vi "load_parameters_csv.vi"(8 "error in (no error)":errorcluster, 10 "Parameter CSV Path":string, 11 "Tags In":string) -> (0 "error out":errorcluster, 1 "Computer Found":bool, 2 "Loaded Params":string[][](array[string]), 3 "Parameters Out":T1)   [LabVIEW 2019]
uses:
  Parameters.ctl
  <vilib>/Utility/file.llb/Read Delimited Spreadsheet (string).vi
panel:
  in  "Parameters":T1
  # "Faux Worm Drawing"
  # "Tracking"
  # "Temporal Calibration"
  # "Stimulus Generation"
  # "Median Filtering"
  # "Experimental Settings"
  # "Camera and Projector Settings"
  # "Faux Worm Drawing"
  # "Tracking"
  # "Temporal Calibration"
  # "Stimulus Generation"
  # "Median Filtering"
  # "Experimental Settings"
  # "Camera and Projector Settings"
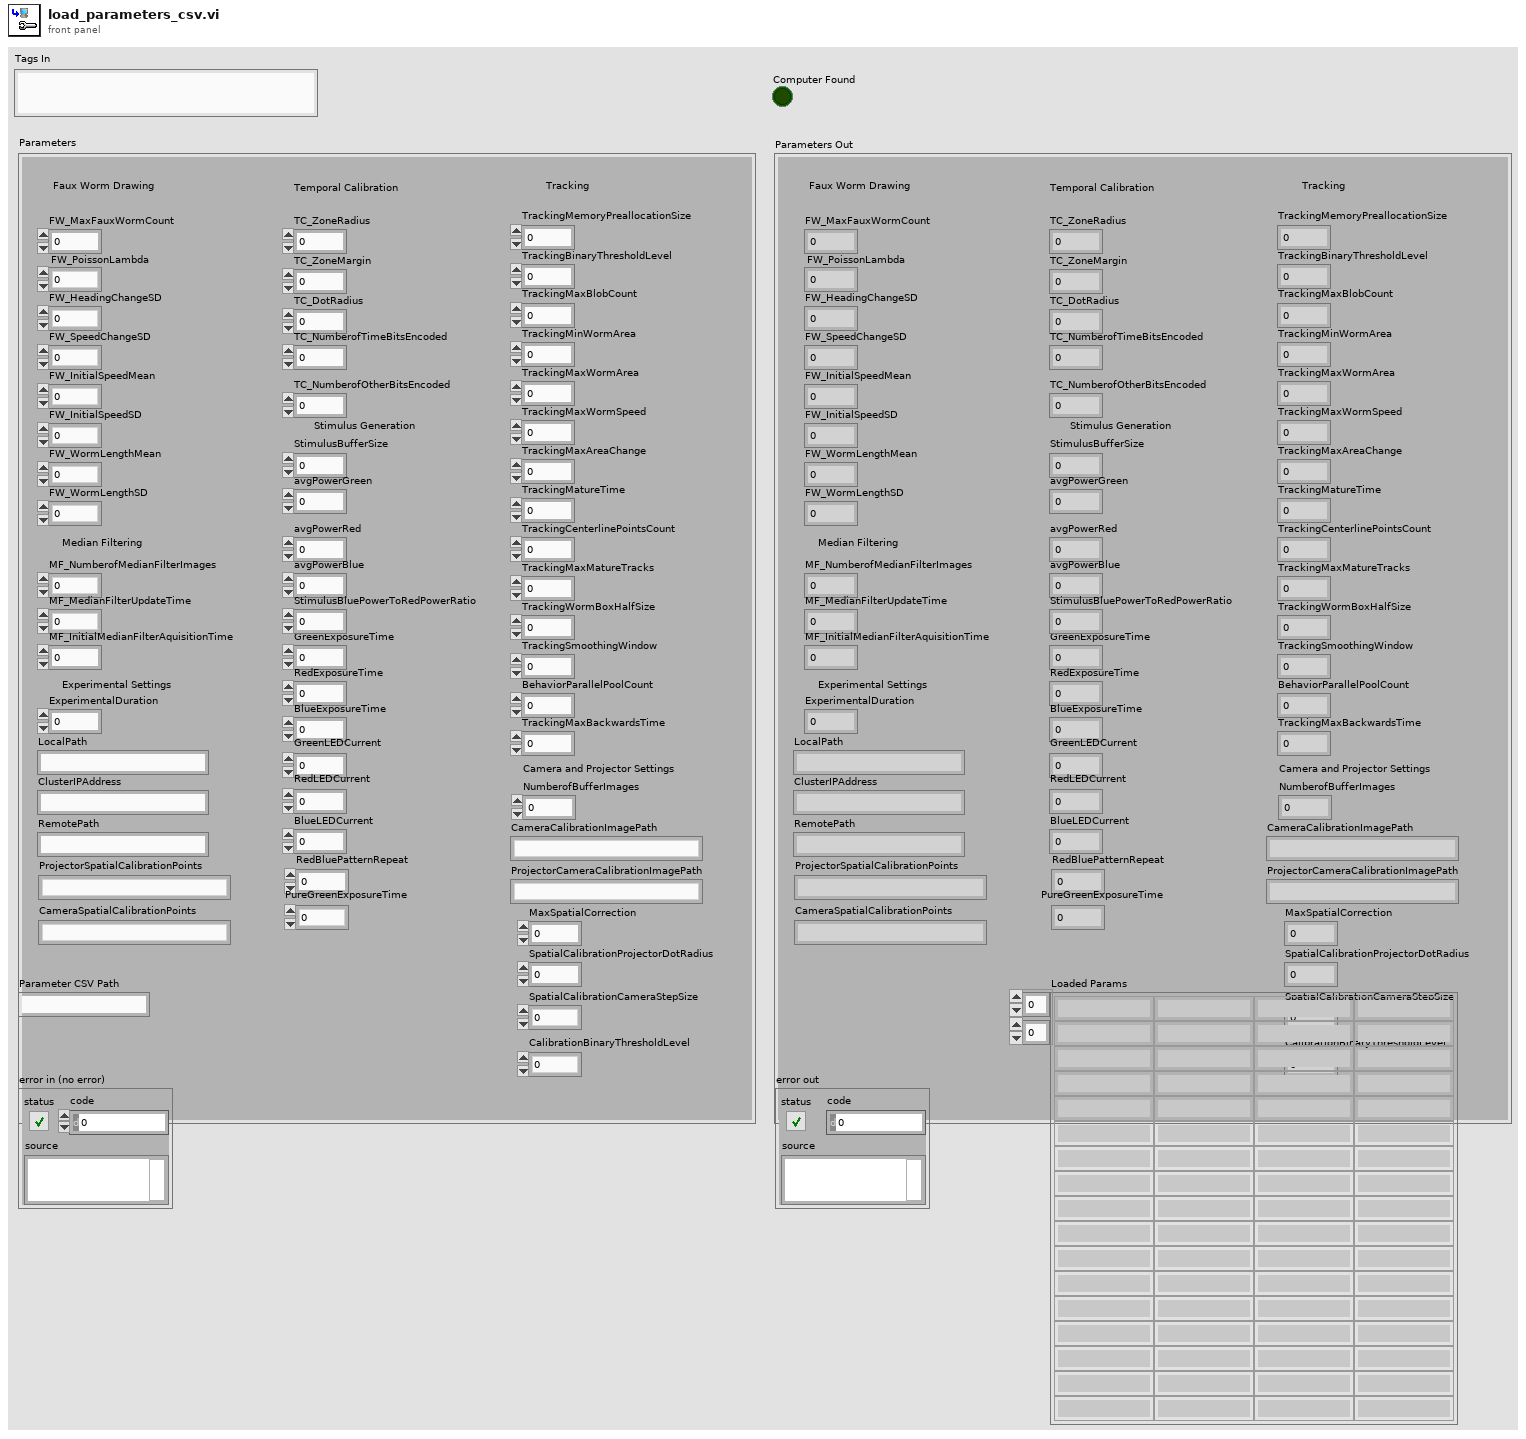
[diagram p1: front panel]
types:
  T1 = typedef "Parameters.ctl" = cluster{"FW_MaxFauxWormCount":i32, "FW_PoissonLambda":dbl, "FW_HeadingChangeSD":dbl, "FW_SpeedChangeSD":dbl, "FW_InitialSpeedMean":dbl, "FW_InitialSpeedSD":dbl, "FW_WormLengthMean":dbl, "FW_WormLengthSD":dbl, "MF_NumberofMedianFilterImages":i32, "MF_MedianFilterUpdateTime":i32, "MF_InitialMedianFilterAquisitionTime":dbl, "ExperimentalDuration":i32, "TC_ZoneRadius":i32, "TC_ZoneMargin":i32, "TC_DotRadius":dbl, "TC_NumberofTimeBitsEncoded":i32, "TC_NumberofOtherBitsEncoded":i32, "NumberofBufferImages":sgl, "CameraCalibrationImagePath":string, "ProjectorCameraCalibrationImagePath":string, "StimulusBufferSize":i32, "TrackingMemoryPreallocationSize":i32, "TrackingBinaryThresholdLevel":sgl, "TrackingMaxBlobCount":i32, "TrackingMinWormArea":dbl, "TrackingMaxWormArea":dbl, "TrackingMaxWormSpeed":dbl, "TrackingMaxAreaChange":dbl, "TrackingMatureTime":i32, "TrackingCenterlinePointsCount":i32, "TrackingMaxMatureTracks":i32, "TrackingWormBoxHalfSize":i32, "TrackingSmoothingWindow":i32, "BehaviorParallelPoolCount":i32, "LocalPath":string, "GreenExposureTime":i32, "RedExposureTime":i32, "BlueExposureTime":i32, "ClusterIPAddress":string, "RemotePath":string, "GreenLEDCurrent":u8, "RedLEDCurrent":u8, "BlueLEDCurrent":u8, "avgPowerGreen":sgl, "avgPowerRed":sgl, "avgPowerBlue":sgl, "StimulusBluePowerToRedPowerRatio":sgl, "TrackingMaxBackwardsTime":i32, "MaxSpatialCorrection":dbl, "ProjectorSpatialCalibrationPoints":string, "SpatialCalibrationProjectorDotRadius":i32, "SpatialCalibrationCameraStepSize":dbl, "CameraSpatialCalibrationPoints":string, "CalibrationBinaryThresholdLevel":dbl, "RedBluePatternRepeat":i32, "PureGreenExposureTime":i32}
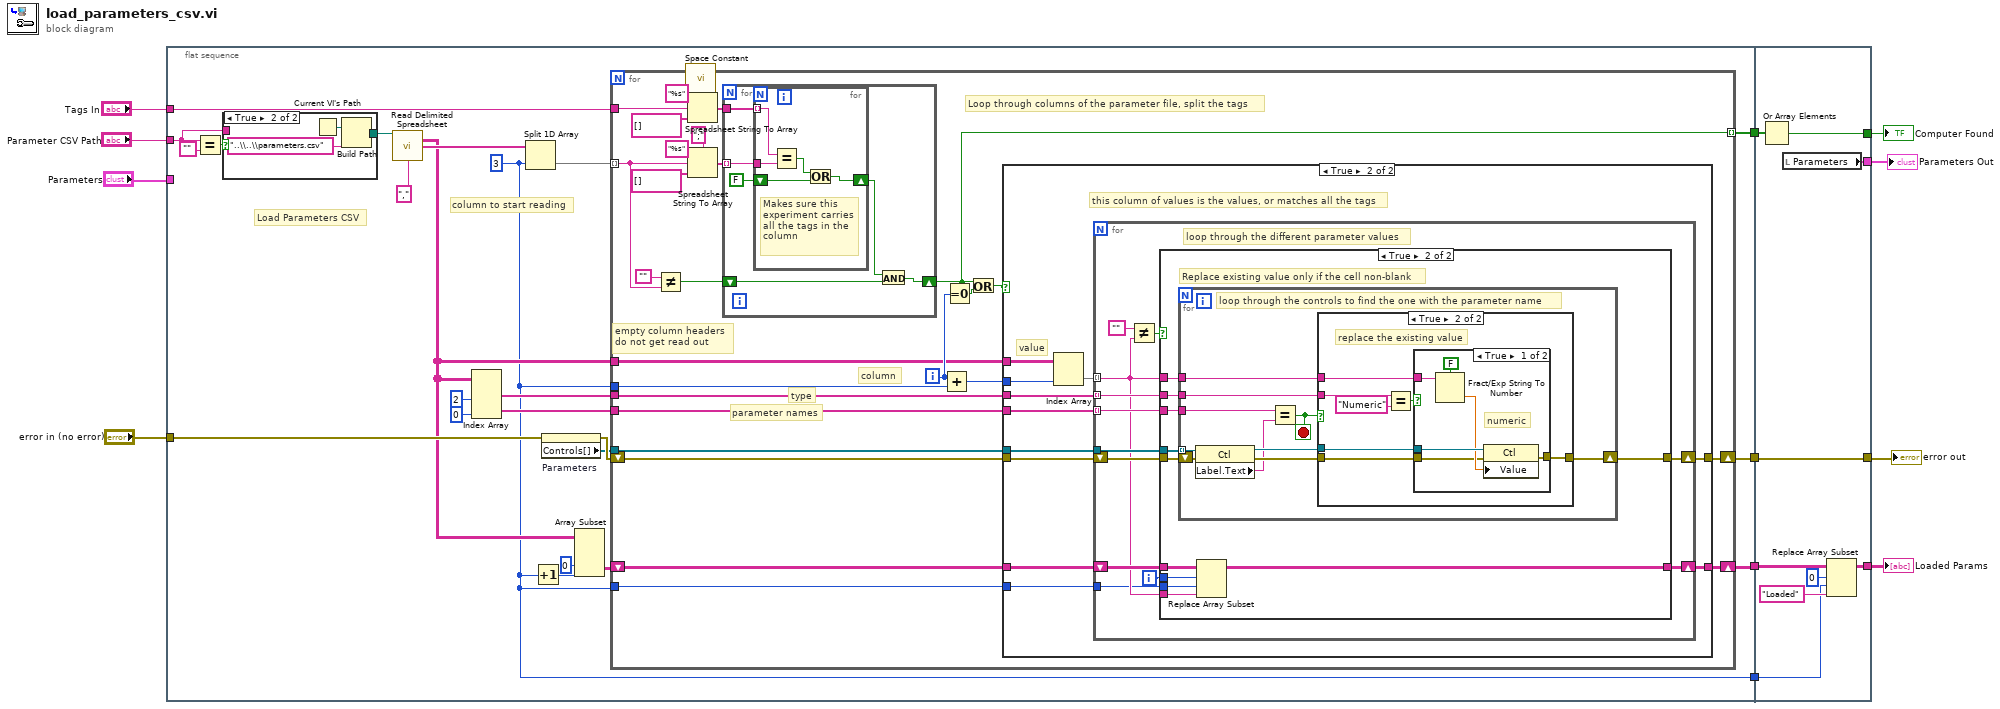
[diagram p0: block diagram]
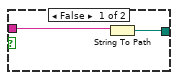
[diagram p2: hidden frame]
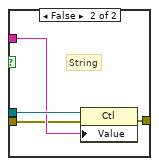
[diagram p6: hidden frame]
diagram:
  n1 = flat-sequence {
    tunnel: "error in (no error)" -> [w25]
    tunnel: [w24] -> w11
    tunnel: "Parameters" -> [_]
    tunnel: "Tags In" -> [w23]
    tunnel: [w19] -> w6
    tunnel: [w17] -> w4
    tunnel: "Parameter CSV Path" -> [w14]
    tunnel: [w13] -> w2
    tunnel: w11 -> [w152]
    tunnel: [w153] -> w10
    tunnel: [w152] -> w9
    tunnel: w6 -> [w149]
    tunnel: [w148] -> w5
    tunnel: w4 -> [w147]
    tunnel: w2 -> [w146]
    tunnel: [w145] -> w1
    frame #0 {
      w17 = 3 ("y")
      # "column to start reading"
      # "Load Parameters CSV"
      n2 = Equal?(x=w14, y="") -> (x = y?=w15:bool)
      n3 = case shown="True" w15 {
        tunnel: [w37 w39] -> w35
        tunnel: w14 -> [w36 _]
        frame False {
          n4 = String To Path(string=w36) -> (path=w37:path)
        }
        frame True {
          n5 = Current VI's Path() -> (path=w40:path)
          n6 = Build Path(base path=w40, name or relative path="..\\..\\parameters.csv") -> (appended path=w39:path)
        }
      }
      n7 = call-poly <vilib>:"Read Delimited Spreadsheet.vi"("file path (dialog if empty)"=w35, "delimiter (\\t)"=",") -> ("all rows"=w18:string[][], "first row"=w27:string[])  [unwired: 8 in, 4 out]
      n8 = Index Array(array=w18, index (col) #1=2 ("disabled index (col)"), index (col) #2=0 ("index (col)")) -> (element #1=w32:string[], element #2=w30:string[])  [unwired: 2 in]
      n9 = Split 1D Array(array=w27, index=w17) -> (second subarray=w26:string[])  [unwired: 1 out]
      n10 = Increment(x=w17) -> (x+1=w21:i32)
      n11 = property on="Parameters" class="Clust (strict)"(error in=w25) -> (error out=w29:errorcluster, "Controls[]"=w28:refnum<vi>[])  [unwired: 1 in, 1 out]
      n12 = Array Subset(array=w18, index (col)=0 ("index"), length (col)=w21) -> (w20:string[][])  [unwired: 2 in]
      n13 = for {
        tunnel: w23 -> [w67]
        tunnel: w26 -> [w46] mode=indexing
        tunnel: w32 -> [w55]
        tunnel: w30 -> [w54]
        tunnel: w18 -> [w53]
        tunnel: w28 -> [w51]
        shift-right: [w49] -> w24
        shift-left: w29 -> [w50]
        tunnel: w17 -> [w48]
        shift-right: [w43] -> w19
        shift-left: w20 -> [w44]
        tunnel: w17 -> [w42]
        tunnel: [w41] -> w13 mode=indexing
        i -> [w58]
        # "empty column headers\ndo not get read out"
        # "type"
        # "parameter names"
        # "column"
        # "Loop through columns of the parameter file, split the tags"
        n14 = Not Equal?(x="", y=w46) -> (x != y?=w45:bool)
        n15 = call <vilib>:"Space Constant.vi"() -> ("String"=w59:string)
        n16 = Spreadsheet String To Array(delimiter (Tab)=w59, format string="%s", spreadsheet string=w67, array type (2D Dbl)=string[] []) -> (array=w64:string[])
        n17 = Spreadsheet String To Array(delimiter (Tab)=";", format string="%s", spreadsheet string=w46, array type (2D Dbl)=string[] []) -> (array=w61:string[])
        n18 = for {
          tunnel: w64 -> [w139]
          tunnel: w61 -> [w138] mode=indexing
          shift-right: [w136] -> w41
          shift-left: w45 -> [w134]
          n19 = for {
            tunnel: w139 -> [w144] mode=indexing
            tunnel: w138 -> [w143]
            shift-right: [w140] -> w135
            shift-left: FALSE -> [w141]
            # "Makes sure this\nexperiment carries\nall the tags in the\ncolumn"
            n20 = Equal?(x=w144, y=w143) -> (x = y?=w142:bool)
            n21 = Or(x=w142, y=w141) -> (x .or. y?=w140:bool)
          }
          n22 = And(x=w135, y=w134) -> (x .and. y?=w136:bool)
        }
        n23 = Add(x=w58, y=w48) -> (x+y=w52:i32)
        n24 = Equal To 0?(x=w58) -> (x = 0?=w57:bool)
        n25 = Or(x=w41, y=w57) -> (x .or. y?=w56:bool)
        n26 = case shown="True" w56 {
          tunnel: w55 -> [_ w77]
          tunnel: w54 -> [_ w76]
          tunnel: w53 -> [_ w80]
          tunnel: w52 -> [_ w79]
          tunnel: w51 -> [_ w75]
          tunnel: w50 -> [w69 w74]
          tunnel: [w69 w73] -> w49
          tunnel: w44 -> [w68 w72]
          tunnel: [w68 w70] -> w43
          tunnel: w42 -> [_ w71]
          frame False {
          }
          frame True {
            # "this column of values is the values, or matches all the tags"
            # "value"
            n27 = Index Array(array=w80, index (col)=w79) -> (element=w78:string[])  [unwired: 1 in]
            n28 = for {
              tunnel: w78 -> [w83] mode=indexing
              tunnel: w77 -> [w89] mode=indexing
              tunnel: w76 -> [w88] mode=indexing
              tunnel: w75 -> [w90]
              shift-right: [w86] -> w73
              shift-left: w74 -> [w87]
              shift-right: [w84] -> w70
              shift-left: w72 -> [w85]
              tunnel: w71 -> [w82]
              i -> [w81]
              # "loop through the different parameter values"
              n29 = Not Equal?(x="", y=w83) -> (x != y?=w91:bool)
              n30 = case shown="True" w91 {
                tunnel: w90 -> [_ w105]
                tunnel: w89 -> [_ w104]
                tunnel: w88 -> [_ w103]
                tunnel: w83 -> [_ w102]
                tunnel: w87 -> [w94 w101]
                tunnel: [w94 w100] -> w86
                tunnel: w85 -> [w93 w99]
                tunnel: [w93 w95] -> w84
                tunnel: w83 -> [_ w96]
                tunnel: w82 -> [_ w98]
                tunnel: w81 -> [_ w97]
                frame False {
                }
                frame True {
                  # "Replace existing value only if the cell non-blank"
                  n31 = for {
                    tunnel: w105 -> [w114] mode=indexing
                    tunnel: w104 -> [w111]
                    tunnel: w103 -> [w115]
                    tunnel: w102 -> [w112]
                    shift-right: [w108] -> w100
                    shift-left: w101 -> [w110]
                    stop <- w107 stop-if-true
                    # "loop through the controls to find the one with the parameter name"
                    n32 = property class="Ctl"(reference=w114, error in=w110) -> (reference out=w113:refnum<vi>, error out=w109:errorcluster, "Label.Text"=w106:string)
                    n33 = Equal?(x=w115, y=w106) -> (x = y?=w107:bool)
                    n34 = case shown="True" w107 {
                      tunnel: w113 -> [_ w123]
                      tunnel: w112 -> [_ w119]
                      tunnel: w111 -> [_ w122]
                      tunnel: w109 -> [w116 w118]
                      tunnel: [w116 w117] -> w108
                      frame False {
                      }
                      frame True {
                        # "replace the existing value"
                        n35 = Equal?(x=w122, y="Numeric") -> (x = y?=w120:bool)
                        n36 = case shown="True" w120 {
                          tunnel: w123 -> [w129 w133]
                          tunnel: w119 -> [w128 w132]
                          tunnel: w118 -> [w126 w130]
                          tunnel: [w125 w131] -> w117
                          frame True {
                            # "numeric"
                            n37 = Fract/Exp String To Number(use system decimal point (T)=FALSE, string=w128) -> (number=w127:dbl)  [unwired: 2 in, 1 out]
                            n38 = property class="Ctl"(reference=w129, error in=w126, "Value"=w127) -> (error out=w125:errorcluster)  [unwired: 1 out]
                          }
                          frame False {
                            # "String"
                            n39 = property class="Ctl"(reference=w133, error in=w130, "Value"=w132) -> (error out=w131:errorcluster)  [unwired: 1 out]
                          }
                        }
                      }
                    }
                  }
                  n40 = Replace Array Subset(array=w99, new element=w96, index (row)=w97, index (col)=w98) -> (w95:string[][])
                }
              }
            }
          }
        }
      }
    }
    frame #1 {
      n41 = Or Array Elements(Boolean array=w146) -> (logical OR=w145:bool)
      n42 = local read "Parameters"() -> (w153:T1)
      n43 = Replace Array Subset(array=w149, new element="Loaded" ("new element/subarray"), index (row)=0 ("disabled index (row)"), index (col)=w147) -> (w148:string[][])
    }
  }
  "Parameters Out" <- w10
  "error out" <- w9
  "Loaded Params" <- w5
  "Computer Found" <- w1
